vi "Fit Spline to Velocity Profile.vi"(9 "X":sgl[](array[numeric]), 10 "positions":dbl[](array[numeric]), 11 "bezier spline":T1) -> (3 "spline adj":cluster{"x":sgl, "y":sgl}[](array[cluster]))   [LabVIEW 2019]
uses:
  Types/Bezier Spline.ctl
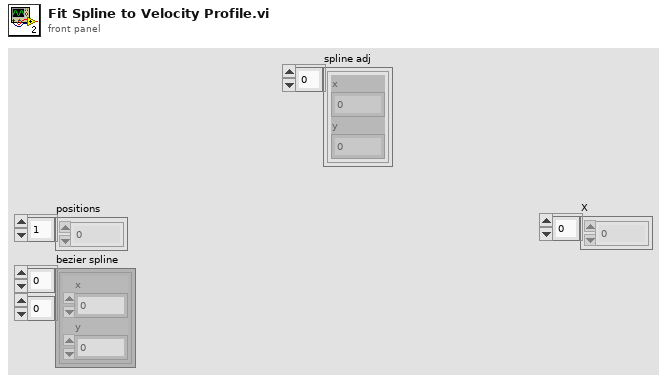
[diagram p1: front panel]
types:
  T1 = typedef "Bezier Spline.ctl" = cluster{"x":sgl, "y":sgl}[][]
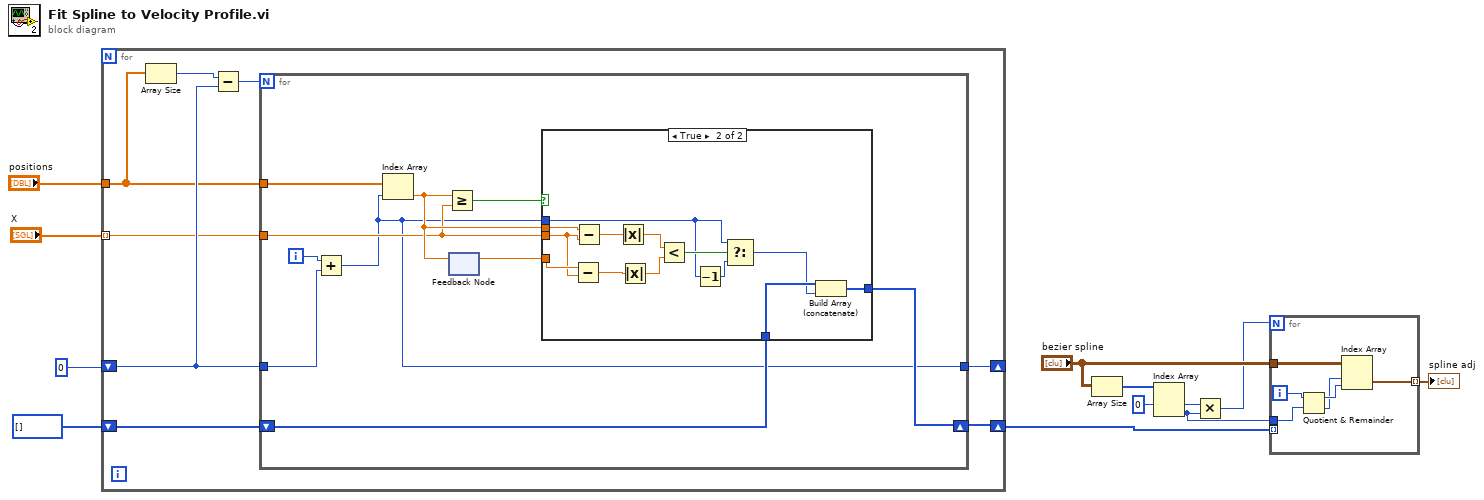
[diagram p0: block diagram]
diagram:
  n1 = for {
    tunnel: "positions" -> [w18]
    tunnel: "X" -> [w16] mode=indexing
    shift-right: [w13] -> _
    shift-left: 0 ("index") -> [w19]
    shift-right: [w14] -> w8
    shift-left: i32[] [] ("appended array") -> [w15]
    n2 = Array Size(array=w18) -> (size(s)=w17:i32)
    n3 = Subtract(x=w17, y=w19) -> (x-y=w20:i32)
    n4 = for {
      N: w20 -> [_]
      tunnel: w18 -> [w30]
      tunnel: w19 -> [w29]
      tunnel: w16 -> [w24]
      shift-right: [w22] -> w14
      shift-left: w15 -> [w23]
      tunnel: [w21] -> w13
      i -> [w28]
      n5 = Add(x=w28, y=w29) -> (x+y=w21:i32)
      n6 = Index Array(array=w30, index=w21) -> (element=w25:dbl)
      n7 = Greater Or Equal?(x=w25, y=w24) -> (x >= y?=w27:bool)
      n8 = feedback-in #1(w25) -> ()
      n9 = feedback #1() -> (w26:dbl)  [unwired: 1 in]
      n10 = case shown="True" w27 {
        tunnel: w26 -> [_ w42]
        tunnel: w25 -> [_ w44]
        tunnel: w24 -> [_ w41]
        tunnel: w21 -> [_ w36]
        tunnel: w23 -> [w31 w34]
        tunnel: [w31 w32] -> w22
        frame False {
        }
        frame True {
          n11 = Subtract(x=w42, y=w41) -> (x-y=w40:dbl)
          n12 = Subtract(x=w44, y=w41) -> (x-y=w43:dbl)
          n13 = Absolute Value(x=w43) -> (abs(x)=w39:dbl)
          n14 = Absolute Value(x=w40) -> (abs(x)=w38:dbl)
          n15 = Less?(x=w39, y=w38) -> (x < y?=w37:bool)
          n16 = Decrement(x=w36) -> (x-1=w35:i32)
          n17 = Select(t=w36, s=w37, f=w35) -> (s? t:f=w33:i32)
          n18 = Build Array (concatenate)(w34, w33) -> (w32:i32[])
        }
      }
    }
  }
  n19 = Array Size(array="bezier spline") -> (size(s)=w6:i32[])
  n20 = Index Array(array=w6, index #1=0 ("index")) -> (element #1=w4:i32, element #2=w2:i32)  [unwired: 1 in]
  n21 = Multiply(x=w4, y=w2) -> (x*y=w3:i32)
  n22 = for {
    N: w3 -> [_]
    tunnel: w8 -> [_] mode=indexing
    tunnel: "bezier spline" -> [w50]
    tunnel: w2 -> [w49]
    tunnel: [w45] -> w1 mode=indexing
    i -> [w48]
    n23 = Quotient & Remainder(x=w48, y=w49) -> (x-y*floor(x/y)=w47:i32, floor(x/y)=w46:i32)
    n24 = Index Array(array=w50, index (row)=w46, index (col)=w47) -> (element=w45:cluster{"x":sgl, "y":sgl})
  }
  "spline adj" <- w1
